vi "newSubvi Safety Check.vi"(0 "VISA In":refnum<visa-resource-name>, 1 "SafetyCheck":T1(ring), 2 "XTarget":i32, 3 "YTarget":i32, 4 "ZTarget":i32) -> (5 "VISA Out":refnum<visa-resource-name>, 6 "Safe":bool, 7 "error out":errorcluster)   [LabVIEW 2012]
doc: "Performs Safety Checks, given the target. Writes to Event Logger."
uses:
  ProSCI Global.vi
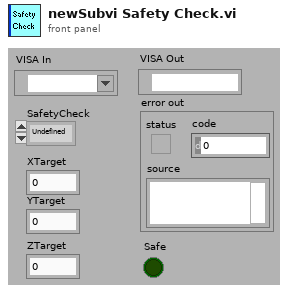
[diagram p1: front panel]
types:
  T1 = enum16{"Undefined", "Focus", "XMin", "YMax", "XY", "Exposure"}
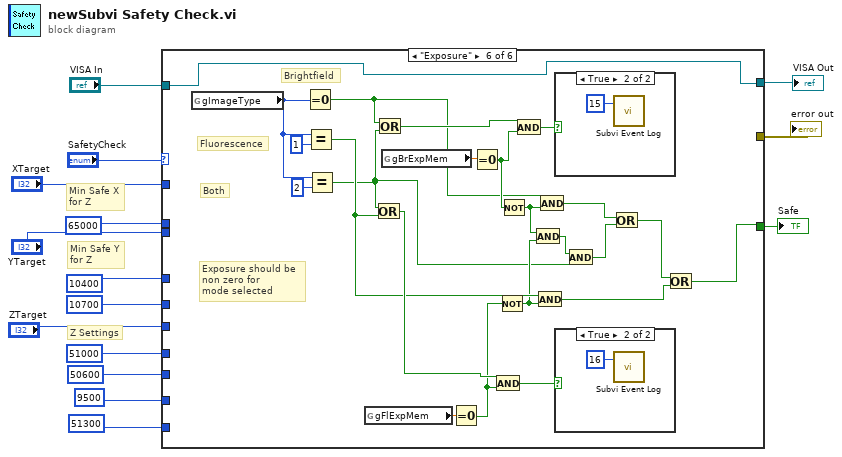
[diagram p0: block diagram]
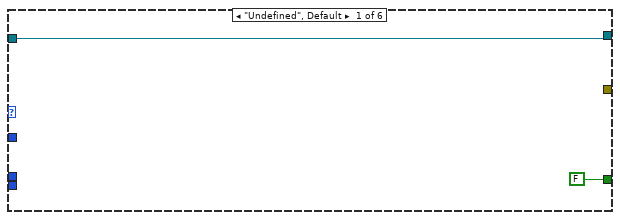
[diagram p2: hidden frame]
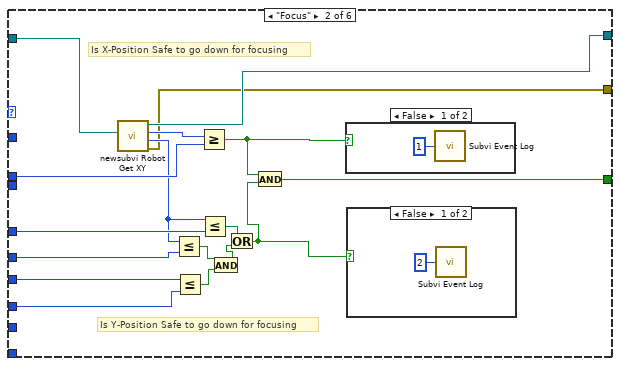
[diagram p3: hidden frame]
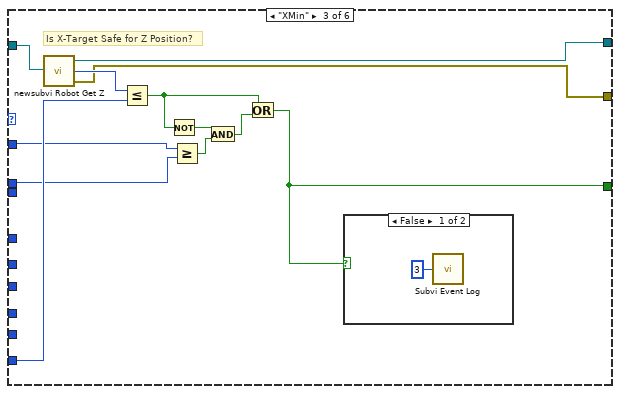
[diagram p6: hidden frame]
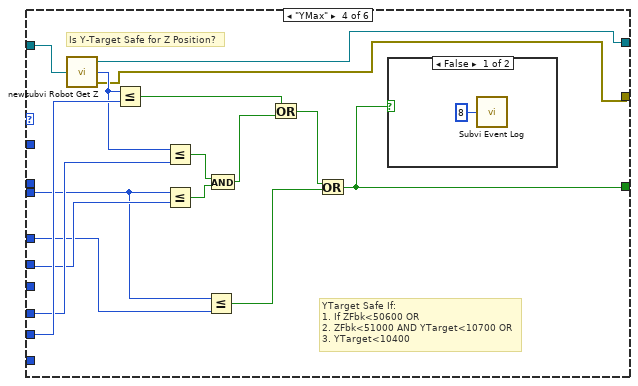
[diagram p8: hidden frame]
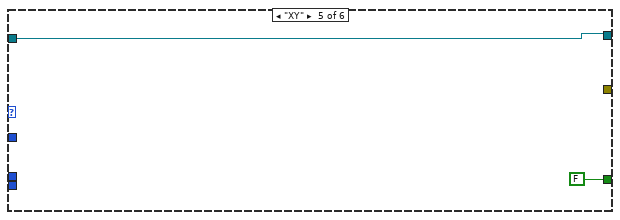
[diagram p10: hidden frame]
diagram:
  # "Z Settings"
  # "Min Safe Y\nfor Z"
  # "Min Safe X\nfor Z"
  n1 = case shown="\"Exposure\"" "SafetyCheck" {
    tunnel: 65000 ("y") -> [_ w33 w41 _ _ _]
    tunnel: 10400 ("y") -> [_ w32 _ w57 _ _]
    tunnel: [FALSE w31 w40 w55 FALSE w70] -> w12
    tunnel: 10700 ("y") -> [_ w28 _ w62 _ _]
    tunnel: "ZTarget" -> [_ w27 _ _ _ _]
    tunnel: 51000 ("y") -> [_ w26 _ w63 _ _]
    tunnel: 9500 ("y") -> [_ _ w45 _ _ _]
    tunnel: "XTarget" -> [_ _ w42 _ _ _]
    tunnel: 50600 ("y") -> [_ _ _ w64 _ _]
    tunnel: "YTarget" -> [_ _ _ w58 _ _]
    tunnel: 51300 ("y") -> [_ _ _ _ _ _]
    tunnel: "VISA In" -> [w16 w20 w39 w52 w67 w69]
    tunnel: [w16 w19 w38 w51 w67 w69] -> w2
    tunnel: [_ w18 w37 w50 _ _] -> w1
    frame "Undefined", Default {
    }
    frame "Focus" {
      # "Is Y-Position Safe to go down for focusing"
      # "Is X-Position Safe to go down for focusing"
      n2 = call "newsubvi Robot Get XY.vi"("VISA In"=w20) -> ("VISA Out"=w19:refnum<visa-resource-name>, "XPosition"=w34:i32, "YPosition"=w29:i32, "error out"=w18:errorcluster)
      n3 = Less Or Equal?(x=w29, y=w28) -> (x <= y?=w24:bool)
      n4 = Less Or Equal?(x=w27, y=w26) -> (x <= y?=w25:bool)
      n5 = Greater Or Equal?(x=w34, y=w33) -> (x >= y?=w30:bool)
      n6 = Less Or Equal?(x=w29, y=w32) -> (x <= y?=w22:bool)
      n7 = And(x=w24, y=w25) -> (x .and. y?=w23:bool)
      n8 = Or(x=w22, y=w23) -> (x .or. y?=w21:bool)
      n9 = And(x=w30, y=w21) -> (x .and. y?=w31:bool)
      n10 = case shown="False" w30 {
        frame False {
          n11 = call "Subvi Event Log.vi"("EventNum"=u32 1) -> ()  [unwired: 1 in]
        }
        frame True {
        }
      }
      n12 = case shown="False" w21 {
        frame False {
          n13 = call "Subvi Event Log.vi"("EventNum"=u32 2) -> ()  [unwired: 1 in]
        }
        frame True {
        }
      }
    }
    frame "XMin" {
      # "Is X-Target Safe for Z Position?"
      n14 = call "newsubvi Robot Get Z.vi"("VISA In"=w39) -> ("VISA Out"=w38:refnum<visa-resource-name>, "ZPosition"=w46:i32, "error out"=w37:errorcluster)
      n15 = Less Or Equal?(x=w46, y=w45) -> (x <= y?=w44:bool)
      n16 = Not(x=w44) -> (.not. x?=w43:bool)
      n17 = Greater Or Equal?(x=w42, y=w41) -> (x >= y?=w48:bool)
      n18 = And(x=w43, y=w48) -> (x .and. y?=w47:bool)
      n19 = Or(x=w44, y=w47) -> (x .or. y?=w40:bool)
      n20 = case shown="False" w40 {
        frame False {
          n21 = call "Subvi Event Log.vi"("EventNum"=u32 3) -> ()  [unwired: 1 in]
        }
        frame True {
        }
      }
    }
    frame "YMax" {
      # "YTarget Safe If:\n1. If ZFbk<50600 OR\n2. ZFbk<51000 AND YTarget<10700 OR\n3. YTarget<10400"
      # "Is Y-Target Safe for Z Position?"
      n22 = call "newsubvi Robot Get Z.vi"("VISA In"=w52) -> ("VISA Out"=w51:refnum<visa-resource-name>, "ZPosition"=w59:i32, "error out"=w50:errorcluster)
      n23 = Less Or Equal?(x=w59, y=w64) -> (x <= y?=w65:bool)
      n24 = Less Or Equal?(x=w59, y=w63) -> (x <= y?=w53:bool)
      n25 = Less Or Equal?(x=w58, y=w62) -> (x <= y?=w60:bool)
      n26 = Less Or Equal?(x=w58, y=w57) -> (x <= y?=w54:bool)
      n27 = And(x=w53, y=w60) -> (x .and. y?=w61:bool)
      n28 = Or(x=w65, y=w61) -> (x .or. y?=w56:bool)
      n29 = Or(x=w56, y=w54) -> (x .or. y?=w55:bool)
      n30 = case shown="False" w55 {
        frame False {
          n31 = call "Subvi Event Log.vi"("EventNum"=u32 8) -> ()  [unwired: 1 in]
        }
        frame True {
        }
      }
    }
    frame "XY" {
    }
    frame "Exposure" {
      # "Exposure should be\nnon zero for\nmode selected"
      # "Both"
      # "Fluorescence"
      # "Brightfield"
      n32 = global read "ProSCI Global.vi" "gImageType"() -> (w91:i8)
      n33 = Equal To 0?(x=w91) -> (x = 0?=w81:bool)
      n34 = Equal?(x=w91, y=i8 1) -> (x = y?=w80:bool)
      n35 = Equal?(x=w91, y=i8 2) -> (x = y?=w75:bool)
      n36 = global read "ProSCI Global.vi" "gFlExpMem"() -> (w83:dbl)
      n37 = Or(x=w75, y=w80) -> (x .or. y?=w84:bool)
      n38 = Or(x=w81, y=w75) -> (x .or. y?=w86:bool)
      n39 = global read "ProSCI Global.vi" "gBrExpMem"() -> (w87:dbl)
      n40 = Equal To 0?(x=w83) -> (x = 0?=w79:bool)
      n41 = Equal To 0?(x=w87) -> (x = 0?=w82:bool)
      n42 = And(x=w84, y=w79) -> (x .and. y?=w85:bool)
      n43 = Not(x=w79) -> (.not. x?=w77:bool)
      n44 = Not(x=w82) -> (.not. x?=w78:bool)
      n45 = And(x=w86, y=w82) -> (x .and. y?=w88:bool)
      n46 = And(x=w78, y=w77) -> (x .and. y?=w76:bool)
      n47 = And(x=w80, y=w77) -> (x .and. y?=w71:bool)
      n48 = And(x=w81, y=w78) -> (x .and. y?=w74:bool)
      n49 = case shown="True" w88 {
        frame False {
        }
        frame True {
          n50 = call "Subvi Event Log.vi"("EventNum"=u32 15) -> ()  [unwired: 1 in]
        }
      }
      n51 = case shown="True" w85 {
        frame False {
        }
        frame True {
          n52 = call "Subvi Event Log.vi"("EventNum"=u32 16) -> ()  [unwired: 1 in]
        }
      }
      n53 = And(x=w76, y=w75) -> (x .and. y?=w73:bool)
      n54 = Or(x=w74, y=w73) -> (x .or. y?=w72:bool)
      n55 = Or(x=w72, y=w71) -> (x .or. y?=w70:bool)
    }
  }
  "Safe" <- w12
  "VISA Out" <- w2
  "error out" <- w1
